vi "节点信息.vi"(0 "node reference":refnum<k20>, 3 "error in (no error)":errorcluster) -> (7 "node reference 2":refnum<k20>, 8 "连接的字符串":string, 10 "error out":errorcluster)   [LabVIEW 2012]
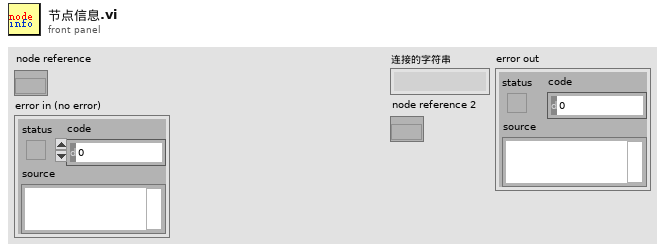
[diagram p1: front panel]
types:
  T1 = typedef "WSN Node Info.ctl" = cluster{"Serial Number":u32, "ID":u32, "Node Type":u16, "Firmware Update State":enum8{"Not Started", "In Progress", "Error", "Done"}, "Firmware Update Percent Complete":u8, "Current Firmware Version":string, "Battery State":u8, "Last Packet Received":timestamp, "Link Quality":enum16{"No Signal", "Poor", "Fair", "Good", "Excellent"}, "Power Supply":enum8{"Battery", "Externally Powered"}, "Network Mode":enum8{"End Device", "Mesh Router"}}
  T2 = enum16{"No Signal", "Poor", "Fair", "Good", "Excellent"}
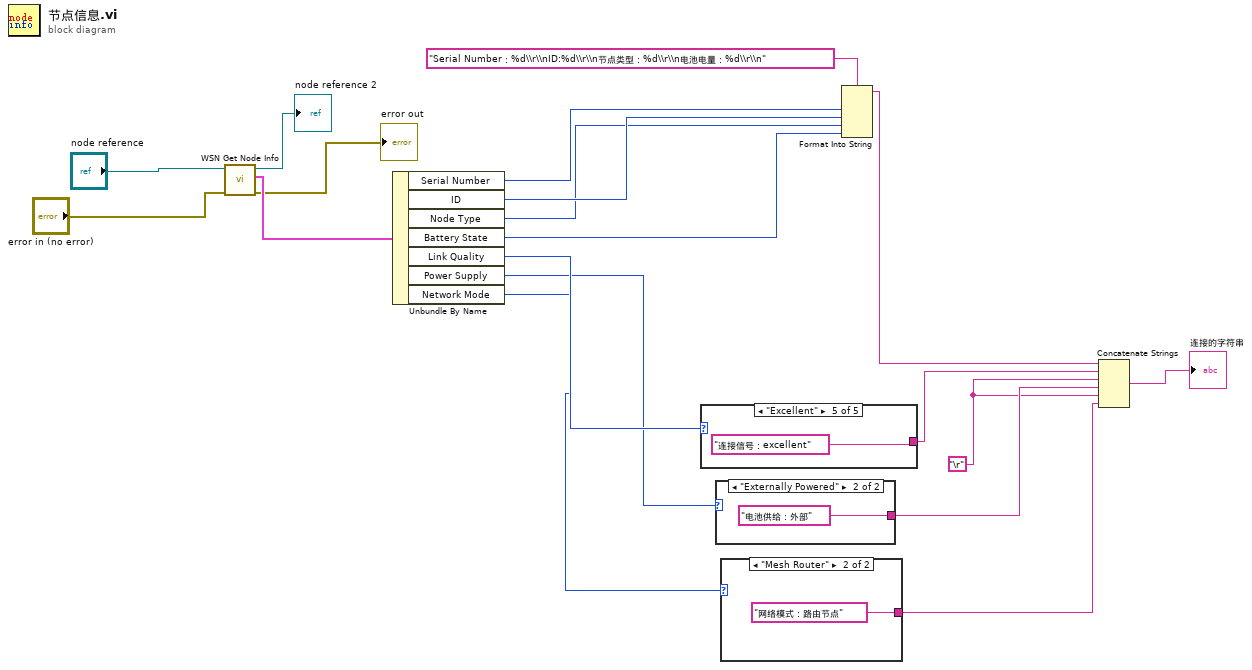
[diagram p0: block diagram]
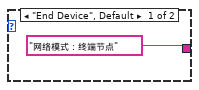
[diagram p2: hidden frame]
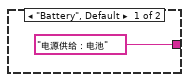
[diagram p3: hidden frame]
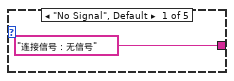
[diagram p4: hidden frame]
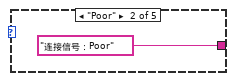
[diagram p5: hidden frame]
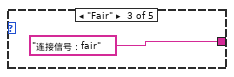
[diagram p6: hidden frame]
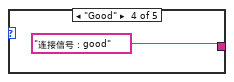
[diagram p7: hidden frame]
diagram:
  w1 = "\r"
  n1 = call <vilib>:"WSN Get Node Info.vi"("error in (no error)"="error in (no error)", "node reference"="node reference") -> ("error out"=→"error out":errorcluster, "node information"=w17:T1, "node reference"=→"node reference 2":refnum<k20>)  [unwired: 7 in]
  n2 = Unbundle By Name(w17) -> ("Serial Number"=w16:u32, "ID"=w15:u32, "Node Type"=w14:u16, "Battery State"=w10:u8, "Link Quality"=w13:T2, "Power Supply"=w12:enum8{"Battery", "Externally Powered"}, "Network Mode"=w11:enum8{"End Device", "Mesh Router"})
  n3 = case shown="\"Excellent\"" w13 {
    tunnel: ["连接信号：无信号" "连接信号：Poor" "连接信号：fair" "连接信号：good" "连接信号：excellent"] -> w7
    frame "No Signal", Default {
    }
    frame "Poor" {
    }
    frame "Fair" {
    }
    frame "Good" {
    }
    frame "Excellent" {
    }
  }
  n4 = case shown="\"Externally Powered\"" w12 {
    tunnel: ["电源供给：电池" "电池供给：外部"] -> w6
    frame "Battery", Default {
    }
    frame "Externally Powered" {
    }
  }
  n5 = case shown="\"Mesh Router\"" w11 {
    tunnel: ["网络模式：终端节点" "网络模式：路由节点"] -> w5
    frame "End Device", Default {
    }
    frame "Mesh Router" {
    }
  }
  n6 = Format Into String(format string="Serial Number：%d\\r\\nID:%d\\r\\n节点类型：%d\\r\\n电池电量：%d\\r\\n" ("格式字符串"), w16, w15, w14, w10) -> (resulting string=w8:string)  [unwired: 2 in, 1 out]
  n7 = Concatenate Strings(w8, w7, w1, w6, w1, w5) -> (→"连接的字符串":string)
